vi "Setup Maps and Queues.vi"(8 "error in (no error)":errorcluster, 11 "WAMP Client in":refnum<class "WAMP Client.lvclass">) -> (0 "error out":errorcluster, 3 "WAMP Client out":refnum<class "WAMP Client.lvclass">)   [LabVIEW 2020, in "wamplv.lvlib" / "WAMP Client.lvclass"]
uses:
  WAMP Client.lvclass
  TypeDef/EVENT payload.ctl
  API/TypeDefs/RESULT payload.ctl
  API/TypeDefs/Combined error.ctl
  API/TypeDefs/WAMP error.ctl
  API/TypeDefs/INVOCATION payload.ctl
  TypeDef/Internal Message.ctl
  TypeDef/Internal Message Type.ctl
  TypeDef/Termination Request.ctl
  WAMP Client.lvclass/WAMP Client.ctl
  TypeDef/Daemon Stopped Event Data.ctl
  TypeDef/Termination Reason Enum.ctl
  TypeDef/Termination Reason.ctl
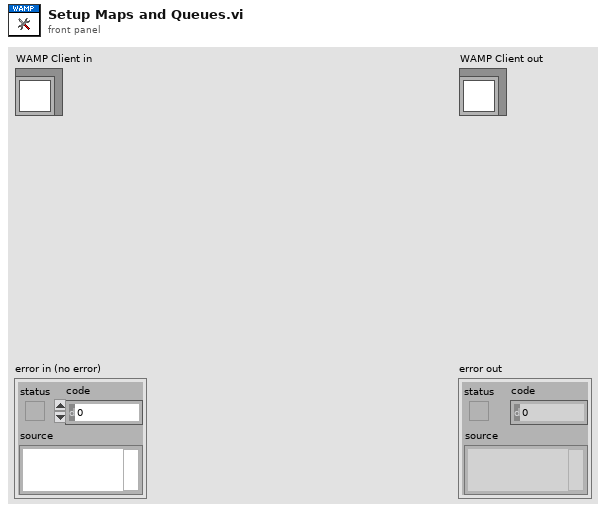
[diagram p1: front panel]
types:
  T1 = typedef "wamplv.lvlib/WAMP Client.lvclass/Termination Request.ctl" = cluster{"Terminate?":bool, "Termination Reason":T2}
  T2 = typedef "wamplv.lvlib/WAMP Client.lvclass/Termination Reason.ctl" = cluster{"Reason":T3, "Reason URI":string, "Message":string}
  T3 = typedef "wamplv.lvlib/WAMP Client.lvclass/Termination Reason Enum.ctl" = enum16{"Goodbye Received", "Abort Received", "Send Goodbye", "Send Abort", "Read Loop Failure", "Write Loop Failure", "Message Loop Failure"}
  T4 = typedef "wamplv.lvlib/WAMP Client.lvclass/Internal Message.ctl" = cluster{"Internal Message Type":T5, "Variant":variant}
  T5 = typedef "wamplv.lvlib/WAMP Client.lvclass/Internal Message Type.ctl" = enum16{"Subscribe", "Handle Subscribed", "Handle Event", "Unsubscribe", "Handle Unsubscribed", "Publish", "Handled Published", "Goodbye", "Handle Goodbye", "Call", "Handle Result", "Register", "Handle Registered", "Unregister", "Handle Unregistered", "Handle Invocation", "Yield", "Error"}
  T6 = typedef "wamplv.lvlib/WAMP Client.lvclass/EVENT payload.ctl" = cluster{"Arguments Payload":string, "ArgumentKw Payload":string, "Topic":string}
  T7 = typedef "wamplv.lvlib/WAMP Client.lvclass/INVOCATION payload.ctl" = cluster{"Arguments":string, "ArgumentKw":string, "Procedure URI":string, "Details":string, "Registration ID":u64, "Request ID":u64}
  T8 = typedef "wamplv.lvlib/WAMP Client.lvclass/Daemon Stopped Event Data.ctl" = cluster{"Error Out":errorcluster, "Termination Reason":T2}
  T9 = typedef "wamplv.lvlib/WAMP Client.lvclass/RESULT payload.ctl" = cluster{"Arguments Payload":string, "ArgumentKw Payload":string, "Topic":string, "Combined Error":T10}
  T10 = typedef "wamplv.lvlib/WAMP Client.lvclass/Combined error.ctl" = cluster{"Error?":bool, "WAMP Error":T11, "Error":errorcluster}
  T11 = typedef "wamplv.lvlib/WAMP Client.lvclass/WAMP error.ctl" = cluster{"Details":string, "ArgumentKw Payload":string, "Error?":bool, "Error URI":string, "Arguments Payload":string}
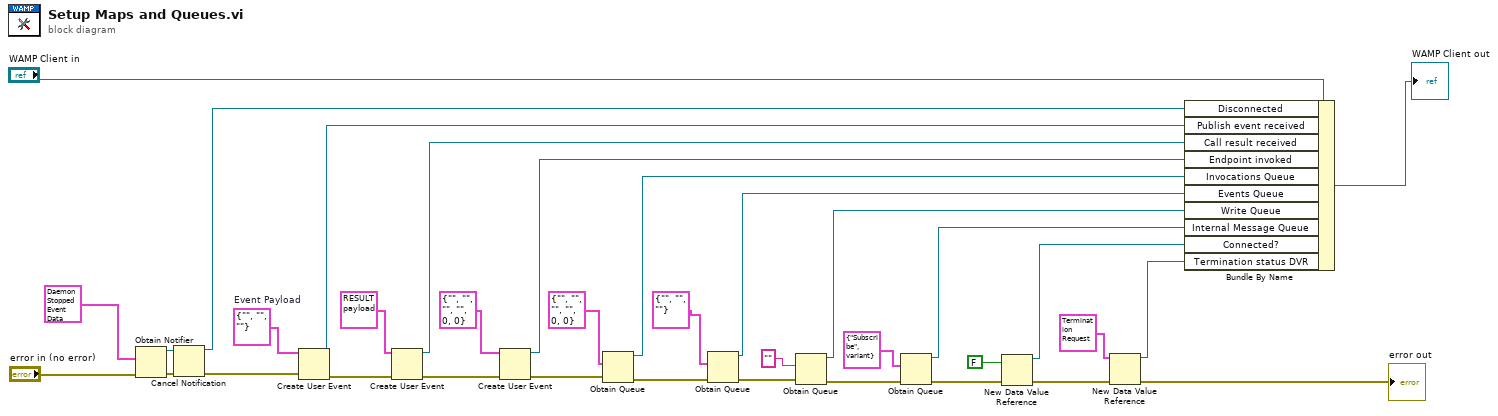
[diagram p0: block diagram]
diagram:
  w35 = T6 {"Arguments Payload"="", "ArgumentKw Payload"="", "Topic"=""}  # Event Payload
  n1 = Obtain Notifier(notification data type=T8 {"Error Out"={"status"=FALSE, "code"=0, "source"=""}, "Termination Reason"={"Reason"=enum."Goodbye Received", "Reason URI"="wamp.error.protocol_violation", "Message"=""}} ("Cluster"), error in (no error)="error in (no error)") -> (notifier out=w4:refnum<notifier>, error out=w3:errorcluster)  [unwired: 2 in, 1 out]
  n2 = Cancel Notification(0:w4, 3:w3) -> (8:w1:refnum<notifier>, 11:w2:errorcluster)  [unwired: 1 out]
  n3 = Create User Event(user event datatype=w35, error in=w2) -> (user event=w34:refnum<user-event>, error out=w31:errorcluster)
  n4 = Create User Event(user event datatype=T9 {"Arguments Payload"="", "ArgumentKw Payload"="", "Topic"="", "Combined Error"={"Error?"=FALSE, "WAMP Error"={"Details"="{}", "ArgumentKw Payload"="", "Error?"=FALSE, "Error URI"="", "Arguments Payload"=""}, "Error"={"status"=FALSE, "code"=0, "source"=""}}} ("RESULT Payload"), error in=w31) -> (user event=w30:refnum<user-event>, error out=w26:errorcluster)
  n5 = Create User Event(user event datatype=T7 {"Arguments"="", "ArgumentKw"="", "Procedure URI"="", "Details"="", "Registration ID"=0, "Request ID"=0} ("INVOCATION payload"), error in=w26) -> (user event=w25:refnum<user-event>, error out=w20:errorcluster)
  n6 = Obtain Queue(element data type=T7 {"Arguments"="", "ArgumentKw"="", "Procedure URI"="", "Details"="", "Registration ID"=0, "Request ID"=0} ("INVOCATION payload"), error in (no error)=w20) -> (queue out=w22:refnum<queue>, error out=w19:errorcluster)  [unwired: 3 in, 1 out]
  n7 = Obtain Queue(element data type=T6 {"Arguments Payload"="", "ArgumentKw Payload"="", "Topic"=""} ("Cluster"), error in (no error)=w19) -> (queue out=w21:refnum<queue>, error out=w12:errorcluster)  [unwired: 3 in, 1 out]
  n8 = Obtain Queue(element data type="", error in (no error)=w12) -> (queue out=w16:refnum<queue>, error out=w18:errorcluster)  [unwired: 3 in, 1 out]
  n9 = Obtain Queue(element data type=T4 {"Internal Message Type"=enum."Subscribe", "Variant"=variant} ("Cluster"), error in (no error)=w18) -> (queue out=w15:refnum<queue>, error out=w10:errorcluster)  [unwired: 3 in, 1 out]
  n10 = New Data Value Reference(data value=FALSE, error in=w10) -> (data value reference=w11:refnum<data-value>, error out=w8:errorcluster)
  n11 = New Data Value Reference(data value=T1 {"Terminate?"=FALSE, "Termination Reason"={"Reason"=enum."Goodbye Received", "Reason URI"="wamp.error.protocol_violation", "Message"=""}} ("Daemon Termination Request"), error in=w8) -> (data value reference=w9:refnum<data-value>, error out=→"error out":errorcluster)
  n12 = Bundle By Name(cluster="WAMP Client in", "Disconnected"=w1, "Publish event received"=w34, "Call result received"=w30, "Endpoint invoked"=w25, "Invocations Queue"=w22, "Events Queue"=w21, "Write Queue"=w16, "Internal Message Queue"=w15, "Connected?"=w11, "Termination status DVR"=w9) -> (→"WAMP Client out":refnum<class "WAMP Client.lvclass">)
